vi "Register For VI Events.vi"(4 "Timeout [ms]":i32=-1, 6 "Timeout Message (to Self)":refnum<class "Message.lvclass">, 7 "Timeout Message Priority (Normal)":T1=enum."Normal", 8 "error in (no error)":errorcluster, 9 "Registration Types":T2[](array[typedef]), 10 "VI Refnum":refnum<vi>, 11 "IEventAggregator In":refnum<class "IEventAggregator.lvclass">) -> (0 "error out":errorcluster, 3 "IEventAggregator Out":refnum<class "IEventAggregator.lvclass">)   [LabVIEW 2015, in "ActorEvents.lvlib" / "IEventAggregator.lvclass"]
uses:
  IEventAggregator.lvclass
  <vilib>/event_ctls.llb/lveventtype.ctl
  <vilib>/ActorFramework/Message/Message.lvclass
  <vilib>/ActorFramework/Message Enqueuer/Message Priority.ctl
  IEventAggregator.lvclass/IEventAggregator.ctl
  EventHandler/VIEventHandler/VIEventHandler.lvclass
  <vilib>/ActorFramework/Message Enqueuer/Message Enqueuer.lvclass
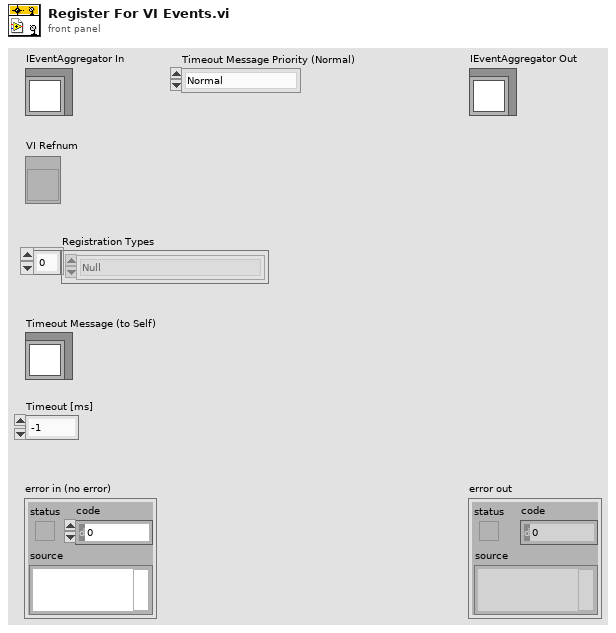
[diagram p1: front panel]
types:
  T1 = typedef "Actor Framework.lvlib/Message Enqueuer.lvclass/Message Priority.ctl" = enum16{"Low", "Normal", "High"}
  T2 = typedef "lveventtype.ctl" = enum32{"Null", "Timeout", "Annotation Menu Selection", "Annotation Menu Selection?", "App Instance Close", "App Instance Close?", "Autoscale Range Change", "Bookmark Info Change", "Cell Edit", "Cell Edit?", "Cursor Grab", "Cursor Grab?", "Cursor Menu Selection", "Cursor Menu Selection?", "Cursor Move", "Cursor Release", "Data Change", "Direction Change", "Display State Change", "Drag Ended", "Drag Enter", "Drag Leave", "Drag Over", "Drag Source Update", "Drag Starting", "Drag Starting?", "Drop", "Exec State Change", "Key Down", "Key Down?", "Key Repeat", "Key Repeat?", "Key Up", "Listbox Double Click", "Menu Activation?", "Menu Selection (App)", "Menu Selection? (App)", "Menu Selection (User)", "Mouse Down", "Mouse Down?", "Mouse Enter", "Mouse Leave", "Mouse Move", "Mouse Up", "Mouse Wheel", "NI Security User Change (App)", "Pane Size", "Panel Close", "Panel Close?", "Panel Resize", "Plot Attribute Change", "Scale Range Change", "Shortcut Menu Activation?", "Shortcut Menu Selection (App)", "Shortcut Menu Selection? (App)", "Shortcut Menu Selection (User)", "Tree Double Click", "Tree Drag", "Tree Drag?", "Tree Drop", "Tree Drop?", "Tree Item Close", "Tree Item Close?", "Tree Item Open", "Tree Item Open?", "User Event", "Value Change"}
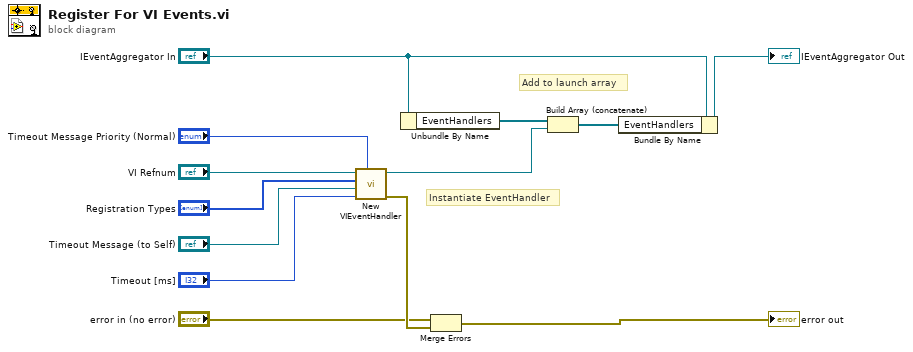
[diagram p0: block diagram]
diagram:
  # "Add to launch array"
  # "Instantiate EventHandler"
  n1 = call "New VIEventHandler.vi"("Timeout Message Priority (Normal)"="Timeout Message Priority (Normal)", "Timeout [ms]"="Timeout [ms]", "Timeout Message"="Timeout Message (to Self)", "Registrations"="Registration Types", "VI Refnum"="VI Refnum") -> ("error out"=w13:errorcluster, "VIEventHandler"=w10:refnum<class "VIEventHandler.lvclass">)  [unwired: 5 in]
  n2 = Unbundle By Name("IEventAggregator In") -> ("EventHandlers"=w12:refnum<class "IEventHandler.lvclass">[])
  n3 = Merge Errors("error in (no error)", w13) -> (→"error out":errorcluster)
  n4 = Build Array (concatenate)(w12, w10) -> (w11:refnum<class "IEventHandler.lvclass">[])
  n5 = Bundle By Name(cluster="IEventAggregator In", "EventHandlers"=w11) -> (→"IEventAggregator Out":refnum<class "IEventAggregator.lvclass">)
